vi "FTW-CodeGen-SetConstantValue.vi"(0 "GObject to Traverse":refnum<vi>, 5 "Constant Label":string="@FTW-CodeGen", 7 "Value":variant, 11 "error in":errorcluster) -> (4 "GObject out":refnum<vi>, 15 "error out":errorcluster)   [LabVIEW 2014]
panel:
  # "Inputs"
  # "Outputs"
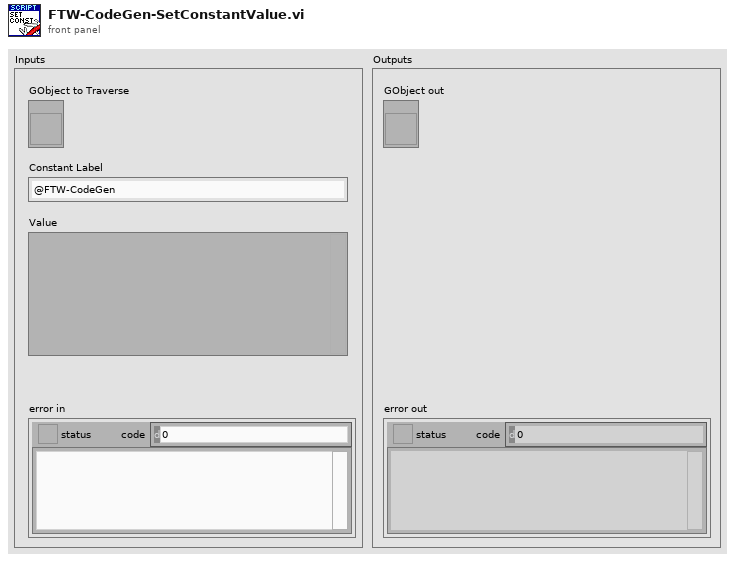
[diagram p1: front panel]
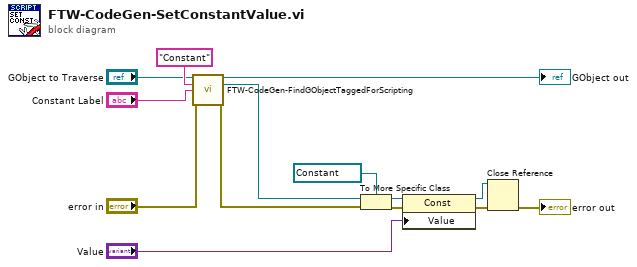
[diagram p0: block diagram]
diagram:
  n1 = call "FTW-CodeGen-FindGObjectTaggedForScripting.vi"("GObject to Traverse"="GObject to Traverse", "Class Name"="Constant", "Label Prefix to uniquely identify node"="Constant Label", "error in"="error in") -> ("GObject to Traverse out"=→"GObject out":refnum<vi>, "GObject"=w13:refnum<vi>, "error out"=w12:errorcluster)  [unwired: 9 in]
  n2 = To More Specific Class(target class=refnum<vi> refnum ("Object"), reference=w13, error in=w12) -> (specific class reference=w11:refnum<vi>, error out=w10:errorcluster)
  n3 = property class="Const"(reference=w11, error in=w10, "Value"="Value") -> (reference out=w8:refnum<vi>, error out=w7:errorcluster)
  n4 = Close Reference(reference=w8, error in (no error)=w7) -> (error out=→"error out":errorcluster)
